vi "Dequeue Data.vi"(8 "error in":errorcluster) -> (0 "error out":errorcluster, 3 "Data":string[][](array[string]))   [LabVIEW 2025, in "Automotive Ethernet Bus Monitor UI.lvlib"]
doc: "Read from the Table Buffer."
uses:
  Automotive Ethernet Bus Monitor UI.lvlib
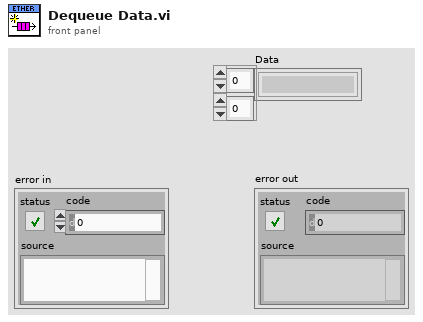
[diagram p1: front panel]
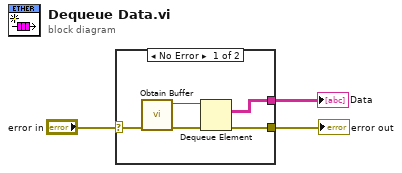
[diagram p0: block diagram]
diagram:
  n1 = case shown="No Error" "error in" {
    selector: "error in" -> [w6 w9]
    tunnel: [w8 w9] -> w2
    tunnel: [w4 _] -> w1
    frame No Error {
      n2 = call "Obtain Buffer.vi"("error in (no error)"=w6) -> ("error out"=w7:errorcluster, "Table Queue"=w5:refnum<queue>)  [unwired: 9 in]
      n3 = Dequeue Element(queue=w5, error in (no error)=w7) -> (element=w4:string[][], error out=w8:errorcluster)  [unwired: 1 in, 2 out]
    }
    frame Error {
    }
  }
  "Data" <- w1
  "error out" <- w2
